vi "保存-定时配置.vi"(8 "error in (no error)":errorcluster caption="错误输入（无错误）", 9 "分别导出?(仅导出定时配置)":bool, 10 "定时配置":T1, 11 "定时器":T2) -> (0 "error out":errorcluster caption="错误输出")   [LabVIEW 2017]
uses:
  <vilib>/Utility/config.llb/Write Key (I32).vi
  <vilib>/Utility/config.llb/Write Key (U32).vi
  <vilib>/Utility/config.llb/Write Key (String).vi
  <vilib>/Utility/config.llb/Write Key (Boolean).vi
  <vilib>/Utility/config.llb/NI_LVConfig.lvlib
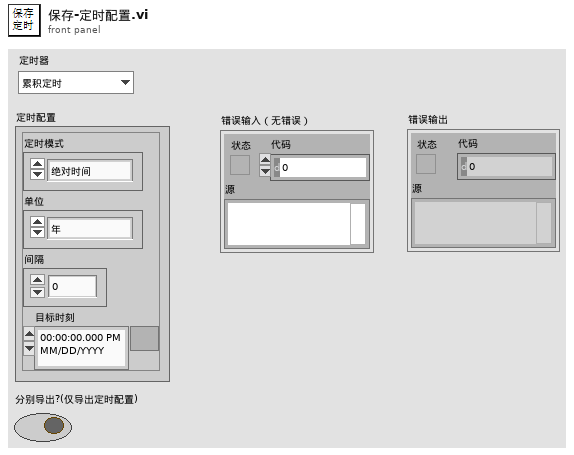
[diagram p1: front panel]
types:
  T1 = typedef "定时配置.ctl" = cluster{"定时模式":enum16{"绝对时间", "相对时间"}, "单位":enum16{"年", "月", "日", "时", "分"}, "间隔":u8, "目标时刻":timestamp}
  T2 = typedef "定时器枚举.ctl" = enum16{"累积定时", "导出定时"}
  T3 = typedef "NI_LVConfig.lvlib/Config Data RefNum.ctl" = refnum<k1>
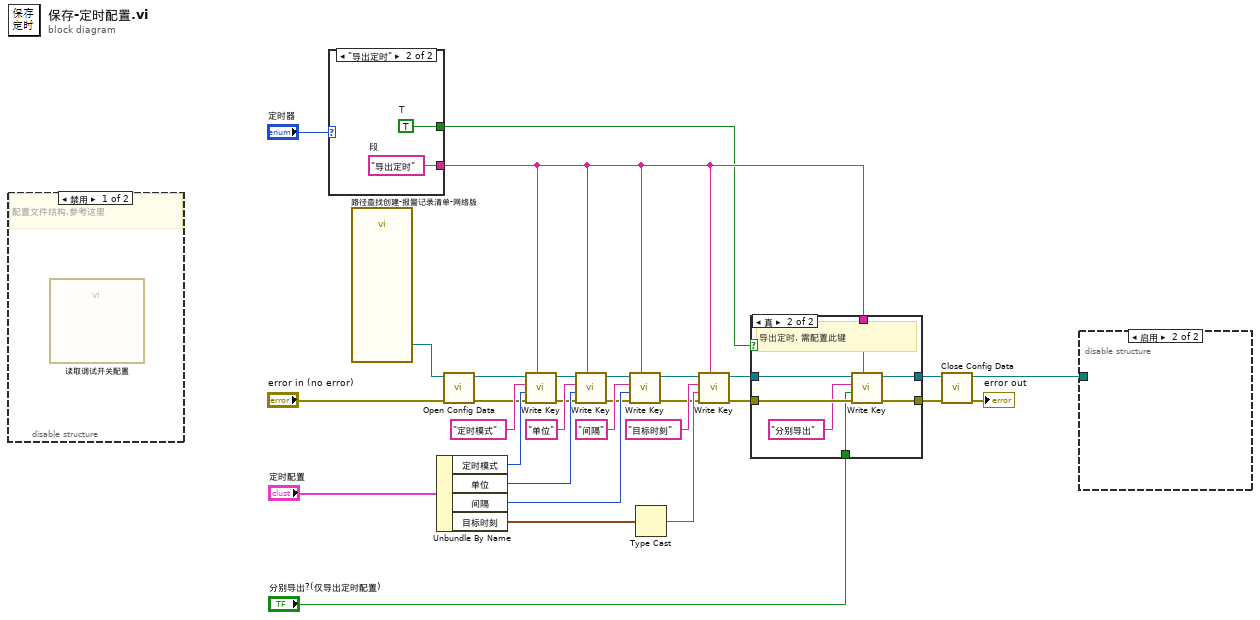
[diagram p0: block diagram]
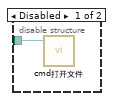
[diagram p2: hidden frame]
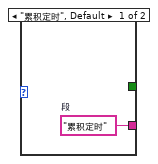
[diagram p5: hidden frame]
diagram:
  n1 = disable-structure shown="禁用" {
    frame Disabled {
      # "配置文件结构,参考这里"
      n2 = call "读取调试开关配置.vi"() -> ()  [unwired: 9 in, 3 out]
    }
    frame Enabled {
    }
  }
  n3 = case shown="\"导出定时\"" "定时器" {
    tunnel: [w31 w33] -> w4
    tunnel: [_ w32] -> w2
    frame "累积定时", Default {
      w31 = "累积定时"  # 段
    }
    frame "导出定时" {
      w32 = TRUE  # T
      w33 = "导出定时"  # 段
    }
  }
  n4 = call "路径查找创建-报警记录清单-网络版.vi"() -> ("配置文件"=w26:path)  [unwired: 2 in, 13 out]
  n5 = Unbundle By Name("定时配置") -> ("定时模式"=w19:enum16{"绝对时间", "相对时间"}, "单位"=w18:enum16{"年", "月", "日", "时", "分"}, "间隔"=w17:u8, "目标时刻"=w16:timestamp)
  n6 = call <vilib>:"Open Config Data.vi"("error in (no error)"="error in (no error)", "configuration file path"=w26) -> ("error out"=w11:errorcluster, "refnum"=w25:T3)  [unwired: 7 in, 1 out]
  n7 = call-poly <vilib>:"Write Key.vi"("section"=w4, "error in (no error)"=w11, "value"=w19, "key"="定时模式" ("section"), "refnum"=w25) -> ("error out"=w12:errorcluster, "refnum out"=w29:T3)  [unwired: 4 in, 1 out]
  n8 = call-poly <vilib>:"Write Key.vi"("section"=w4, "error in (no error)"=w12, "value"=w18, "key"="单位" ("section"), "refnum"=w29) -> ("error out"=w10:errorcluster, "refnum out"=w27:T3)  [unwired: 4 in, 1 out]
  n9 = call-poly <vilib>:"Write Key.vi"("section"=w4, "error in (no error)"=w10, "value"=w17, "key"="间隔" ("section"), "refnum"=w27) -> ("error out"=w9:errorcluster, "refnum out"=w28:T3)  [unwired: 4 in, 1 out]
  n10 = Type Cast(x=w16) -> (*(type *) &x=w15:string)  [unwired: 1 in]
  n11 = call-poly <vilib>:"Write Key.vi"("section"=w4, "error in (no error)"=w9, "value"=w15, "key"="目标时刻" ("section"), "refnum"=w28) -> ("error out"=w8:errorcluster, "refnum out"=w6:T3)  [unwired: 4 in, 1 out]
  n12 = case shown="真" w2 {
    tunnel: w8 -> [w34 w42]
    tunnel: [w34 w41] -> w7
    tunnel: w6 -> [w35 w40]
    tunnel: [w35 w39] -> w5
    tunnel: w4 -> [_ w38]
    tunnel: "分别导出?(仅导出定时配置)" -> [_ w36]
    frame False {
      # "累积定时, 跳过"
    }
    frame True {
      # "导出定时, 需配置此键"
      n13 = call-poly <vilib>:"Write Key.vi"("section"=w38, "error in (no error)"=w42, "value"=w36, "key"="分别导出" ("section"), "refnum"=w40) -> ("error out"=w41:errorcluster, "refnum out"=w39:T3)  [unwired: 4 in, 1 out]
    }
  }
  n14 = call <vilib>:"Close Config Data.vi"("error in (no error)"=w7, "refnum"=w5) -> ("error out"=→"error out":errorcluster, "file path"=w1:path)  [unwired: 8 in]
  n15 = disable-structure shown="启用" {
    disable-tunnel: w1 -> [w43 _]
    frame Disabled {
      n16 = call "cmd打开文件.vi"("文件路径"=w43) -> ()  [unwired: 10 in, 1 out]
    }
    frame Enabled {
    }
  }
